vi "Connection Handlers.vi"(9 "Connection Handler Map":T1, 11 "Processing In":refnum<class "Processing.lvclass">) -> (1 "Close?":bool, 3 "HTTP Server.lvlib:Processing":refnum<class "Processing.lvclass">)   [LabVIEW 2020, in "HTTP Server.lvlib" / "Server.lvclass"]
uses:
  Server.lvclass
  Processing/Processing.lvclass
  Connection Handler Map.ctl
  Priority.ctl
  Connection Handler/Connection Handler.lvclass
  Processing Step.ctl
  Processing/Processing.lvclass/Processing.ctl
  HTTP TCP Client/HTTP TCP Client.lvclass
  C:/dev/lv20CE/relink/lv-stream/stream/Endpoint/Endpoint.lvclass
  Server.lvclass/Server.ctl
  RequestTraceLog/RequestTraceLog.lvclass
  HTTP Server.lvlib
  C:/dev/lv20CE/relink/lv-http-server/HTTP Server/Connection Handler/Connection Handler.lvclass
  C:/dev/lv20CE/relink/lv-http-server/HTTP Server/Handler/Handler.lvclass
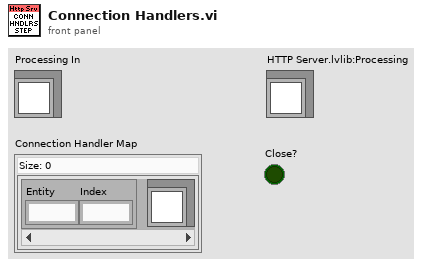
[diagram p1: front panel]
types:
  T1 = typedef "HTTP Server.lvlib/Connection Handler Map.ctl" = map{T2, refnum<class "Connection Handler.lvclass">}
  T2 = typedef "HTTP Server.lvlib/Priority.ctl" = cluster{"Entity":u16, "Index":u16}
  T3 = typedef "HTTP Server.lvlib/Processing Step.ctl" = enum16{"Connection", "Request", "Routing", "Controller Init", "Controller", "Response", "Complete", "Exception"}
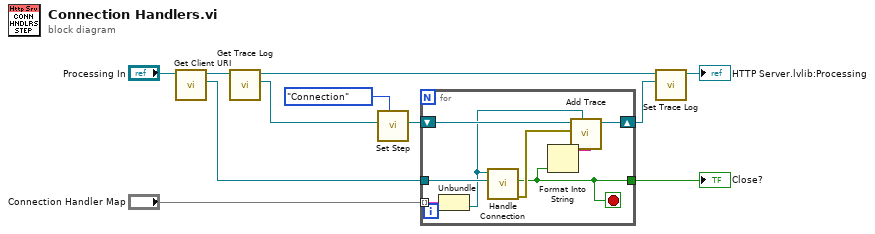
[diagram p0: block diagram]
diagram:
  n1 = call "Get Client URI.vi"("Processing in"="Processing In") -> ("Client URI"=w1:refnum<class "URI.lvclass">, "Processing out"=w2:refnum<class "Processing.lvclass">)  [unwired: 9 in]
  n2 = call "Get Trace Log.vi"("Processing in"=w2) -> ("Trace Log"=w7:refnum<class "RequestTraceLog.lvclass">, "Processing out"=w6:refnum<class "Processing.lvclass">)  [unwired: 9 in]
  n3 = call "Set Step.vi"("Processing Step"=Processing_Step."Connection", "RequestTraceLog in"=w7) -> ("RequestTraceLog out"=w8:refnum<class "RequestTraceLog.lvclass">)  [unwired: 9 in]
  n4 = for {
    tunnel: "Connection Handler Map" -> [w19] mode=indexing
    tunnel: w1 -> [w18]
    tunnel: [w13] -> w10
    shift-right: [w16] -> w5
    shift-left: w8 -> [w17]
    stop <- w13 stop-if-true
    n5 = Unbundle(w19) -> ("Handler"=w14:refnum<class "Connection Handler.lvclass">)  [unwired: 1 out]
    n6 = call-dynamic "Handle Connection.vi"("Client URI"=w18, "Connection Handler in"=w14) -> ("error out"=w15:errorcluster, "Close?"=w13:bool)  [unwired: 8 in]
    n7 = Format Into String(w13) -> (resulting string=w12:string)  [unwired: 3 in, 1 out]
    n8 = call "Add Trace.vi"("Info"=w12, "LabVIEW Object"=w14, "error in (no error)"=w15, "RequestTraceLog in"=w17) -> ("RequestTraceLog out"=w16:refnum<class "RequestTraceLog.lvclass">)  [unwired: 6 in, 1 out]
  }
  "Close?" <- w10
  n9 = call "Set Trace Log.vi"("Trace Log"=w5, "Processing in"=w6) -> ("Processing out"=→"HTTP Server.lvlib:Processing":refnum<class "Processing.lvclass">)  [unwired: 9 in]
